vi "HTS_WELL_TO_PLATE.vi"(1 "Well Array":T1[](array[typedef])) -> (0 "Array":bool[][](array[boolean]))   [LabVIEW 2009]
uses:
  HTS_WELL.ctl
  HTS_COLUMN.ctl
  HTS_ROW.ctl
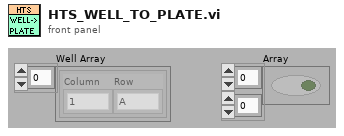
[diagram p1: front panel]
types:
  T1 = typedef "HTS_WELL.ctl" = cluster{"Column":T2, "Row":T3}
  T2 = typedef "HTS_COLUMN.ctl" = enum16{"1", "2", "3", "4", "5", "6", "7", "8", "9", "10", "11", "12"}
  T3 = typedef "HTS_ROW.ctl" = enum16{"A", "B", "C", "D", "E", "F", "G", "H"}
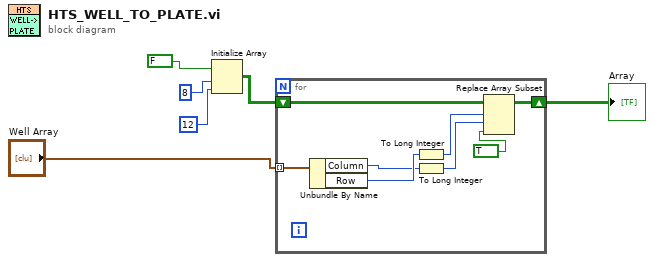
[diagram p0: block diagram]
diagram:
  n1 = Initialize Array(FALSE ("Boolean"), 8 ("dimension size"), 12 ("dimension size")) -> (w4:bool[][])
  n2 = for {
    tunnel: "Well Array" -> [w13] mode=indexing
    shift-right: [w7] -> w5
    shift-left: w4 -> [w14]
    n3 = Unbundle By Name(w13) -> ("Column"=w8:T2, "Row"=w9:T3)
    n4 = To Long Integer(number=w9) -> (32bit integer=w11:i32)
    n5 = To Long Integer(number=w8) -> (32bit integer=w10:i32)
    n6 = Replace Array Subset(array=w14, new element=TRUE ("new element/subarray"), index (row)=w11, index (col)=w10) -> (w7:bool[][])
  }
  "Array" <- w5
